vi "load 16bit image fr file to array.vi"(3 "error in (no error)":errorcluster, 4 "Image Name":string="loaded image", 5 "Dispose images":bool, 6 "File Path":path) -> (0 "error out":errorcluster, 1 "Image":T2(plugin-control), 2 "Intensity Graph":u16[][](graph))   [LabVIEW 2013]
panel:
  in  "File Options":T1 {"Optional Max Value" format="%.2f"; "Optional Min Value" format="%.2f"; "File Data Type" items=["1 bit", "2 bits", "4 bits", "8 bits", "16 bits (unsigned)", "16 bits (signed)", "16 bits (RGB chunky)", "24 bits (RGB chunky)", "24 bits (RGB planar)", "32 bits (unsigned)", "32 bits (signed)", "32 bits (RGB chunky)", "32 bits (float)", "48 bits (Complex 2x24 int)", "64 bits (Complex 2x32 float)", "32 bits (HSL)"]; "Read Raw File" items=["Don't Read Raw File ", "Read Raw File"]}
  # "Y:\\100TWdata\\Y2010\\Apr\\10_0427\\scans\\Scan000\\SideView"
  # "Z:\\TREXResources\\HexapodPosition\\capentranceZLocation\\8SideView.png"
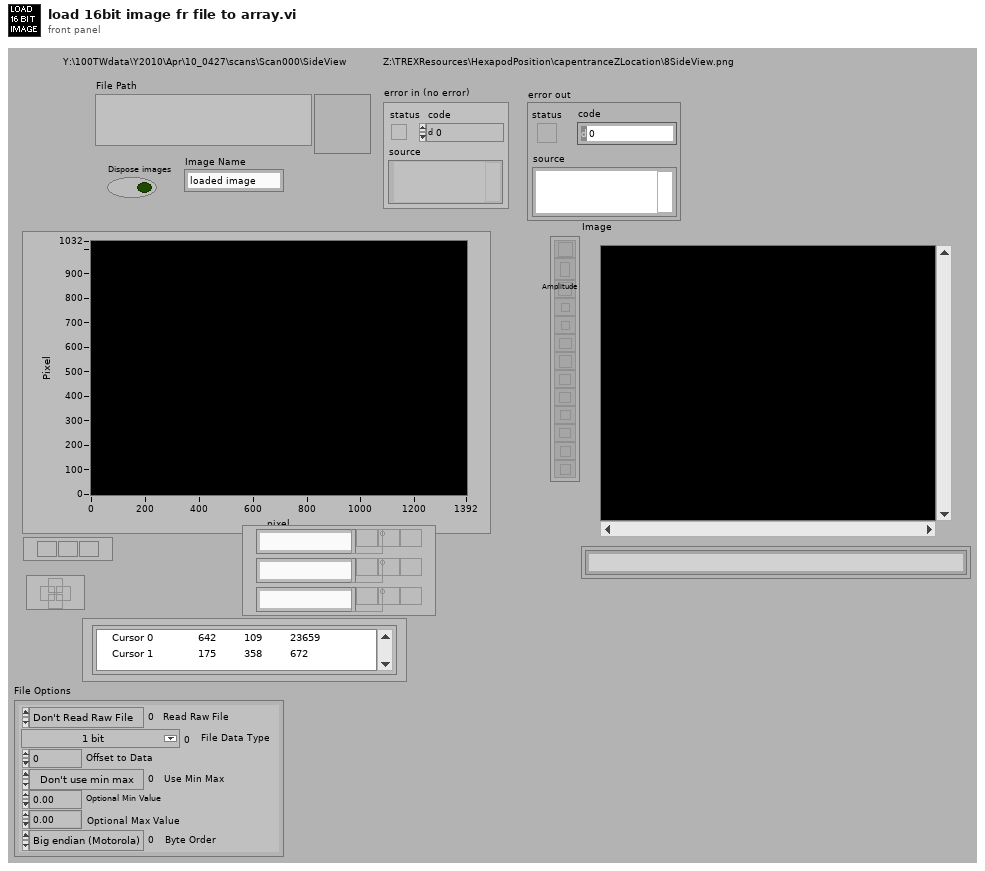
[diagram p1: front panel]
types:
  T1 = cluster{"Read Raw File":i32, "File Data Type":u32, "Offset to Data":i32, "Use Min Max":enum32{"Don't use min max", "Use file values", "Use optional values"}, "Optional Min Value":sgl, "Optional Max Value":sgl, "Byte Order":enum32{"Big endian (Motorola)", "Little endian (Intel)"}}
  T2 = typedef "IMAQ Image.ctl" = refnum<image>
  T3 = typedef "Image Type" = u32
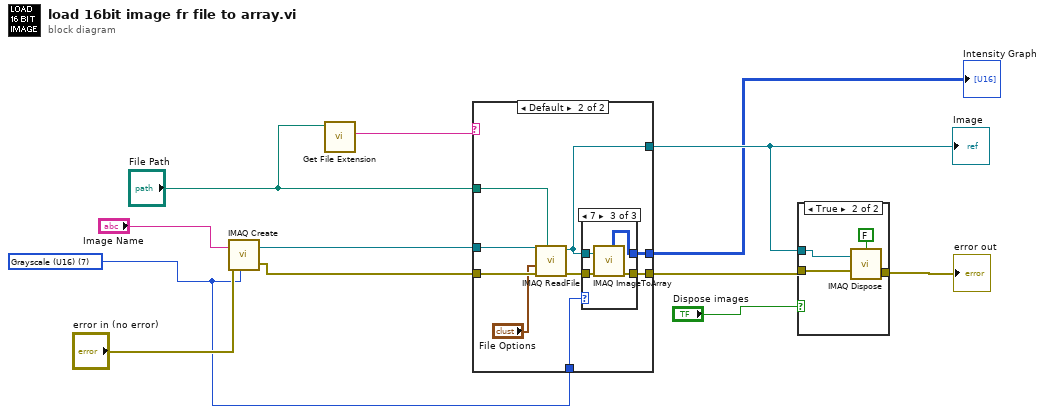
[diagram p0: block diagram]
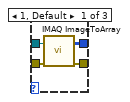
[diagram p3: hidden frame]
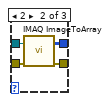
[diagram p4: hidden frame]
diagram:
  w1 = T3 7 items=["Grayscale (U8)", "Grayscale (I16)", "Grayscale (SGL)", "Complex (CSG)", "RGB (U32)", "HSL (U32)", "RGB (U64)", "Grayscale (U16)"] ("Image Type")
  n1 = call "IMAQ Create"("Image Name"="Image Name", "Image Type"=w1, "error in (no error)"="error in (no error)") -> ("New Image"=w11:T2, "error out"=w9:errorcluster)  [unwired: 1 in, 1 out]
  n2 = call <vilib>:"Get File Extension.vi"("file"="File Path") -> ("lowercase file extension"=w2:string)  [unwired: 1 in, 9 out]
  n3 = case shown="Default" w2 {
    tunnel: w11 -> [_ w21]
    tunnel: "File Path" -> [_ w20]
    tunnel: w9 -> [_ w19]
    tunnel: [_ w17] -> w6
    tunnel: [_ w16] -> w5
    tunnel: [_ w15] -> w4
    tunnel: w1 -> [_ w13]
    frame "fits" {
    }
    frame Default {
      n4 = call "IMAQ ReadFile"("File Path"=w20, "error in (no error)"=w19, "File Options"="File Options", "Image"=w21) -> ("error out"=w18:errorcluster, "Image Out"=w17:T2)  [unwired: 1 in, 5 out]
      n5 = case shown="7" w13 {
        tunnel: w18 -> [w25 w29 w33]
        tunnel: w17 -> [w24 w28 w32]
        tunnel: [w23 w27 w31] -> w16
        tunnel: [w22 w26 w30] -> w15
        frame 1, Default {
          n6 = call "IMAQ ImageToArray"("error in (no error)"=w25, "Image"=w24) -> ("error out"=w23:errorcluster, "Image Pixels (I16)"=w22:i16[][])  [unwired: 1 in, 4 out]
        }
        frame 2 {
          n7 = call "IMAQ ImageToArray"("error in (no error)"=w29, "Image"=w28) -> ("error out"=w27:errorcluster, "Image Pixels (I16)"=w26:i16[][])  [unwired: 1 in, 4 out]
        }
        frame 7 {
          n8 = call "IMAQ ImageToArray"("error in (no error)"=w33, "Image"=w32) -> ("Image Pixels (U16)"=w30:u16[][], "error out"=w31:errorcluster)  [unwired: 1 in, 4 out]
        }
      }
    }
  }
  "Image" <- w6
  "Intensity Graph" <- w4
  n9 = case shown="True" "Dispose images" {
    tunnel: w5 -> [w34 w38]
    tunnel: [w34 w37] -> w8
    tunnel: w6 -> [_ w36]
    frame False {
    }
    frame True {
      n10 = call "IMAQ Dispose"("All Images? (No)"=FALSE, "Image"=w36, "error in (no error)"=w38) -> ("error out"=w37:errorcluster)  [unwired: 3 out]
    }
  }
  "error out" <- w8
